vi "Call.vi"(4 "ArgumentsKw":string, 6 "Arguments":string, 7 "Timeout (ms)":i32=500, 8 "Error in":errorcluster, 9 "Options":string, 10 "Topic URI":string, 11 "WAMP Client in":refnum<class "WAMP Client.lvclass">) -> (0 "Error out":errorcluster, 1 "ArgumentKw Payload":string, 2 "Arguments Payload":string, 3 "WAMP Client out":refnum<class "WAMP Client.lvclass">, 5 "WAMP Error":T1={"Details"="{}", "ArgumentKw Payload"="{}", "Error?"=FALSE, "Error URI"="", "Arguments Payload"=""})   [LabVIEW 2020, in "wamplv.lvlib" / "WAMP Client.lvclass"]
uses:
  WAMP Client.lvclass
  TypeDefs/WAMP error.ctl
  TypeDefs/RESULT payload.ctl
  TypeDefs/Combined error.ctl
  <vilib>/Utility/error.llb/Error Cluster From Error Code.vi
  <vilib>/ErrorRing/Error Ring.xnode
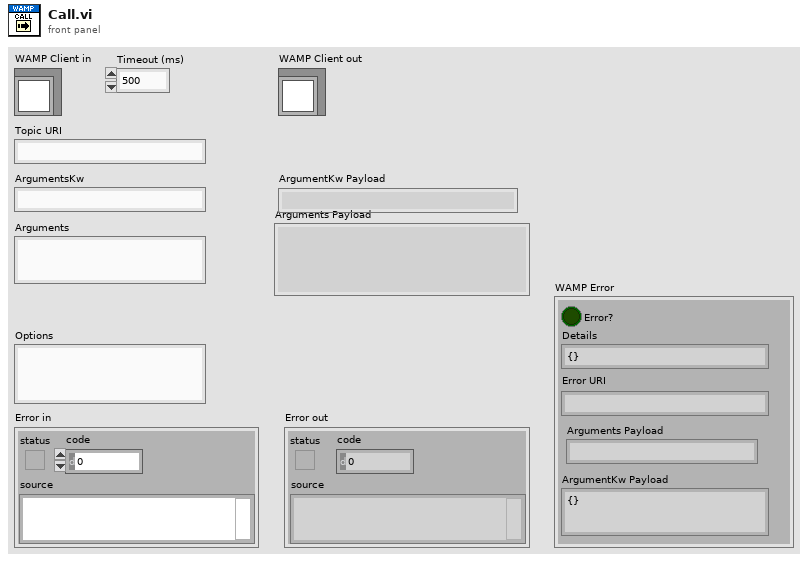
[diagram p1: front panel]
types:
  T1 = typedef "wamplv.lvlib/WAMP Client.lvclass/WAMP error.ctl" = cluster{"Details":string, "ArgumentKw Payload":string, "Error?":bool, "Error URI":string, "Arguments Payload":string}
  T2 = typedef "wamplv.lvlib/WAMP Client.lvclass/RESULT payload.ctl" = cluster{"Arguments Payload":string, "ArgumentKw Payload":string, "Topic":string, "Success?":bool, "Combined Error":T3}
  T3 = typedef "wamplv.lvlib/WAMP Client.lvclass/Combined error.ctl" = cluster{"Error?":bool, "WAMP Error":T1, "Error":errorcluster}
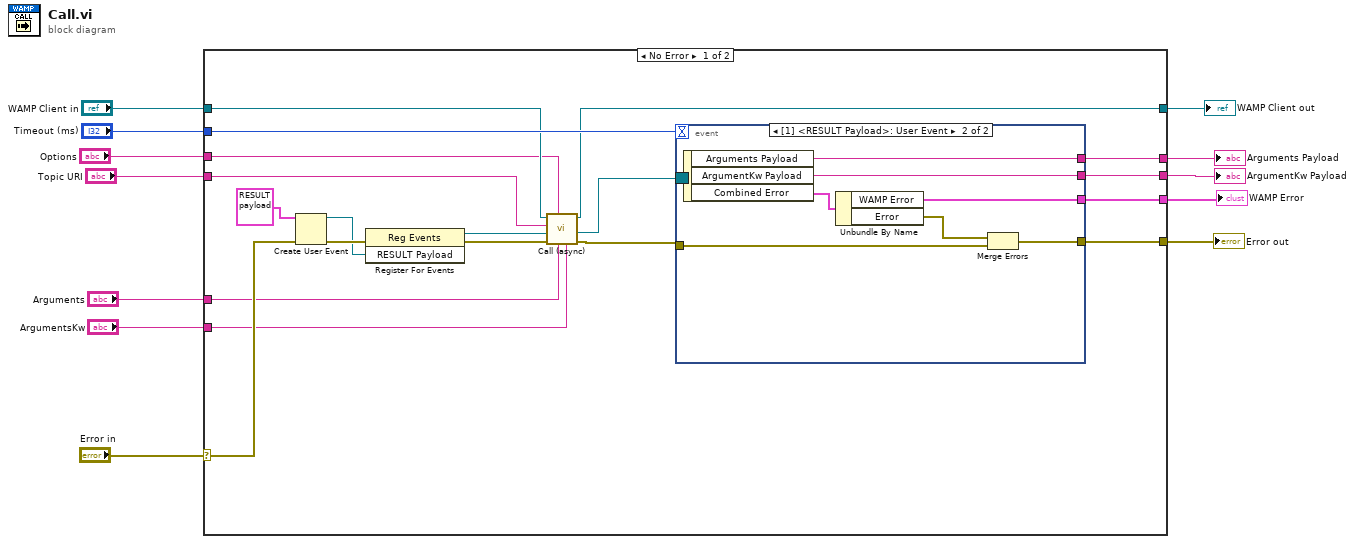
[diagram p0: block diagram]
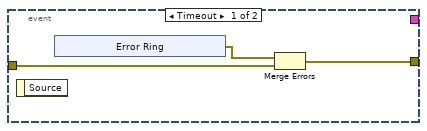
[diagram p2: hidden frame]
diagram:
  n1 = case shown="No Error" "Error in" {
    selector: "Error in" -> [w29 w47]
    tunnel: [w19 w47] -> w11
    tunnel: [w25 w46] -> w9
    tunnel: "WAMP Client in" -> [w24 w46]
    tunnel: "Topic URI" -> [w17 _]
    tunnel: "Arguments" -> [w21 _]
    tunnel: "ArgumentsKw" -> [w20 _]
    tunnel: "Timeout (ms)" -> [w26 _]
    tunnel: [w28 _] -> w1
    tunnel: [w27 _] -> w4
    tunnel: [w18 _] -> w3
    tunnel: "Options" -> [w14 _]
    frame No Error {
      n2 = Create User Event(user event datatype=T2 {"Arguments Payload"="", "ArgumentKw Payload"="", "Topic"="", "Success?"=FALSE, "Combined Error"={"Error?"=FALSE, "WAMP Error"={"Details"="{}", "ArgumentKw Payload"="", "Error?"=FALSE, "Error URI"="", "Arguments Payload"=""}, "Error"={"status"=FALSE, "code"=0, "source"=""}}} ("RESULT Payload"), error in=w29) -> (user event=w22:refnum<user-event>, error out=w23:errorcluster)
      n3 = register-events(error in=w23, w22) -> (reference out=w13:refnum<event-registration>, error out=w16:errorcluster)  [unwired: 1 in]
      n4 = call "Call (async).vi"("ArgumentsKw"=w20, "Arguments"=w21, "Options"=w14, "error in (no error)"=w16, "Call Result Event"=w22, "Topic URI"=w17, "WAMP Client in"=w24) -> ("error out"=w15:errorcluster, "WAMP Client out"=w25:refnum<class "WAMP Client.lvclass">)  [unwired: 3 in]
      n5 = event shown="[1] <RESULT Payload>: User Event" {
        selector: w13 -> [_ _]
        dyn-events: _ -> [_ _]
        timeout: w26 -> [_ _]
        tunnel: [_ w45] -> w28
        tunnel: [_ w44] -> w27
        tunnel: w15 -> [w31 w40]
        tunnel: [w32 w43] -> w19
        tunnel: [_ w39] -> w18
        event Timeout {
          n6 = event-data() -> ()  [unwired: 1 in, 1 out]
          n7 = xnode "Error Ring"() -> ("error out"=w33:errorcluster)
          n8 = Merge Errors(w33, w31) -> (w32:errorcluster)
        }
        event User Event {
          n9 = event-data() -> ("Arguments Payload"=w45:string, "ArgumentKw Payload"=w44:string, "Combined Error"=w41:T3)  [unwired: 1 in]
          n10 = Unbundle By Name(w41) -> ("WAMP Error"=w39:T1, "Error"=w42:errorcluster)
          n11 = Merge Errors(w42, w40) -> (w43:errorcluster)
        }
      }
    }
    frame Error {
    }
  }
  "Error out" <- w11
  "WAMP Client out" <- w9
  "Arguments Payload" <- w1
  "ArgumentKw Payload" <- w4
  "WAMP Error" <- w3
